vi "AM MODULATION.vi"() -> ()   [LabVIEW 2017]
panel:
  out "MODULATION":dynamicdata(graph)
  out "CARRIER":dynamicdata(graph)
  out "MESSAGE":dynamicdata(graph)
  in  "Ac":dbl caption="Phase"
  in  "Am":dbl caption="Phase"
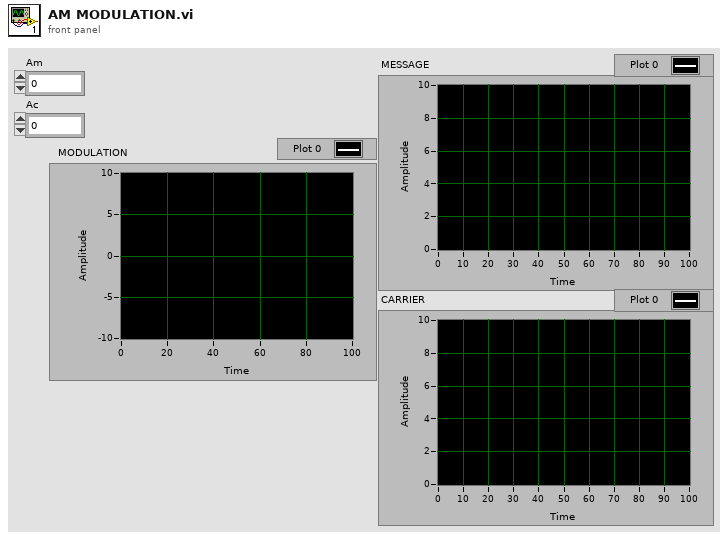
[diagram p1: front panel]
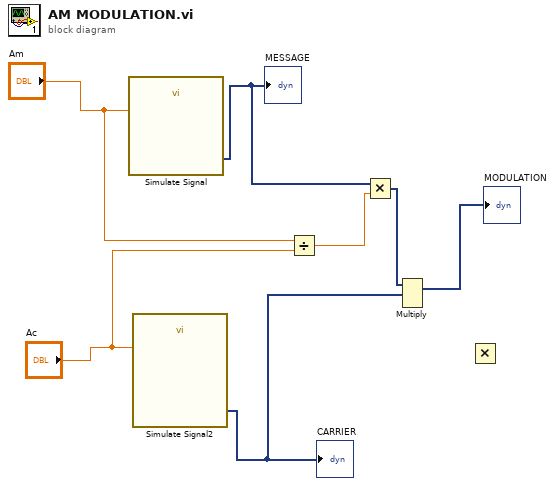
[diagram p0: block diagram]
diagram:
  n1 = call "Simulate Signal"("Phase"="Am") -> ("MESSAGE"=w5:dynamicdata)  [unwired: 13 in, 1 out]
  "MESSAGE" <- w5
  n2 = call "Simulate Signal2"("Phase"="Ac") -> ("CARRIER"=w2:dynamicdata)  [unwired: 13 in, 1 out]
  "CARRIER" <- w2
  n3 = Divide(x="Am", y="Ac") -> (x/y=w4:dbl)
  n4 = Multiply(x=w5, y=w4) -> (x*y=w3:dynamicdata)
  n5 = Multiply(1:w2, 2:w3) -> (0:→"MODULATION":dynamicdata)  [unwired: 1 in, 1 out]
  n6 = Multiply() -> ()  [unwired: 2 in, 1 out]
